vi "FX33.vi"(11 "Variables and Memory in":T1 {"GFX" format="%02x"}) -> (3 "Variables and Memory out":T1 {"GFX" format="%02x"})   [LabVIEW 2021]
uses:
  Controls/ClusterF.ctl
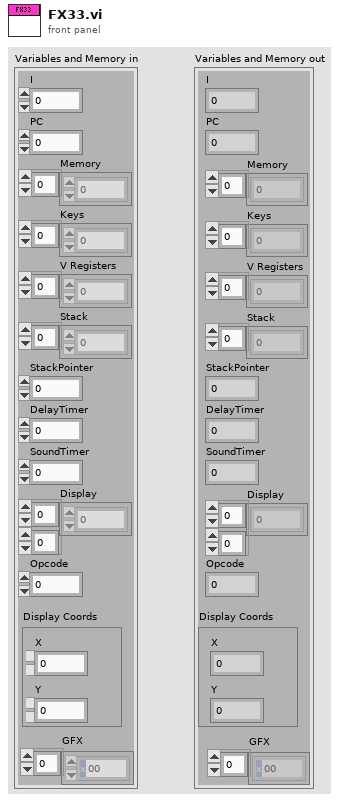
[diagram p1: front panel]
types:
  T1 = typedef "ClusterF.ctl" = cluster{"I":u16, "PC":u16, "Memory":u8[], "Keys":u8[], "V Registers":u8[], "Stack":u16[], "StackPointer":u16, "DelayTimer":u8, "SoundTimer":u8, "Display":u8[][], "Opcode":u16, "Display Coords":cluster{"X":u8, "Y":u8}, "GFX":u8[]}
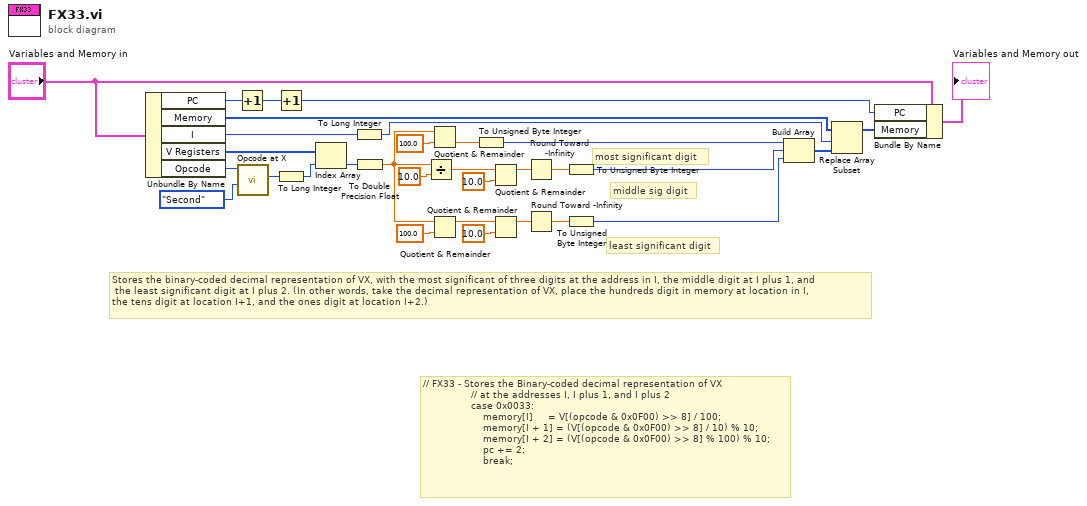
[diagram p0: block diagram]
diagram:
  # "// FX33 - Stores the Binary-coded decimal representation of VX\n                // at the addresses I, I plus 1, and I plus 2\n                case 0x0033:\n                    memory[I]     = V[(opcode & 0x0F00) >> 8] / 100;\n                    memory[I + 1] = (V[(opcode & 0x0F00) >> 8] / 10) % 10;\n                    memory[I + 2] = (V[(opcode & 0x0F00) >> 8] % 100) % 10;\n                    pc += 2;\n                    break;"
  # "middle sig digit"
  # "Stores the binary-coded decimal representation of VX, with the most significant of three digits at the address in I, the middle digit at I plus 1, and\n the least significant digit at I plus 2. (In other words, take the decimal representation of VX, place the hundreds digit in memory at location in I, \nthe tens digit at location I+1, and the ones digit at location I+2.)"
  # "least significant digit"
  # "most significant digit"
  n1 = Unbundle By Name("Variables and Memory in") -> ("PC"=w3:u16, "Memory"=w24:u8[], "I"=w25:u16, "V Registers"=w8:u8[], "Opcode"=w6:u16)
  n2 = Increment(x=w3) -> (x+1=w4:u16)
  n3 = call "Opcode at X.vi"("X Position"=enum16{"First", "Second", "Third", "Fourth"}."Second", "Opcode"=w6) -> ("Opcode at X Position (U8)"=w9:u8)  [unwired: 9 in]
  n4 = Increment(x=w4) -> (x+1=w5:u16)
  n5 = To Long Integer(number=w9) -> (32bit integer=w10:i32)
  n6 = Index Array(array=w8, index=w10) -> (element=w32:u8)
  n7 = To Long Integer(number=w25) -> (32bit integer=w26:i32)
  n8 = To Double Precision Float(number=w32) -> (double precision float=w18:dbl)
  n9 = Divide(x=w18, y=10.0) -> (x/y=w14:dbl)
  n10 = Quotient & Remainder(x=w18, y=100.0) -> (floor(x/y)=w12:dbl)  [unwired: 1 out]
  n11 = Quotient & Remainder(x=w18, y=100.0) -> (x-y*floor(x/y)=w22:dbl)  [unwired: 1 out]
  n12 = To Unsigned Byte Integer(number=w12) -> (unsigned 8bit integer=w27:u8)
  n13 = Quotient & Remainder(x=w14, y=10.0) -> (x-y*floor(x/y)=w16:dbl)  [unwired: 1 out]
  n14 = Quotient & Remainder(x=w22, y=10.0) -> (x-y*floor(x/y)=w23:dbl)  [unwired: 1 out]
  n15 = Round Toward -Infinity(1:w16) -> (0:w17:dbl)
  n16 = Round Toward -Infinity(1:w23) -> (0:w21:dbl)
  n17 = To Unsigned Byte Integer(number=w17) -> (unsigned 8bit integer=w28:u8)
  n18 = To Unsigned Byte Integer(number=w21) -> (unsigned 8bit integer=w29:u8)
  n19 = Build Array(w27, w28, w29) -> (w30:u8[])
  n20 = Replace Array Subset(array=w24, new element=w30, index=w26) -> (w31:u8[])
  n21 = Bundle By Name(cluster="Variables and Memory in", "PC"=w5, "Memory"=w31) -> (→"Variables and Memory out":T1)
